vi "SetPoint.vi"(0 "Input":dbl, 1 "IAd(AI2)":dbl, 3 "I+(BI2)":bool, 4 "I-(BI1)":bool, 5 "Igrd(AI1)":dbl, 6 "ILL(AI3)":dbl=1.0, 7 "error in":errorcluster, 8 "ULL(AI4)":dbl=1.0, 9 "SetP Grad":dbl, 12 "IC(BI3)":bool, 14 "SetP UL":dbl, 15 "SetP LL":dbl) -> (23 "Output (AO1)":dbl, 27 "error out":errorcluster)   [LabVIEW 2022 SP3]
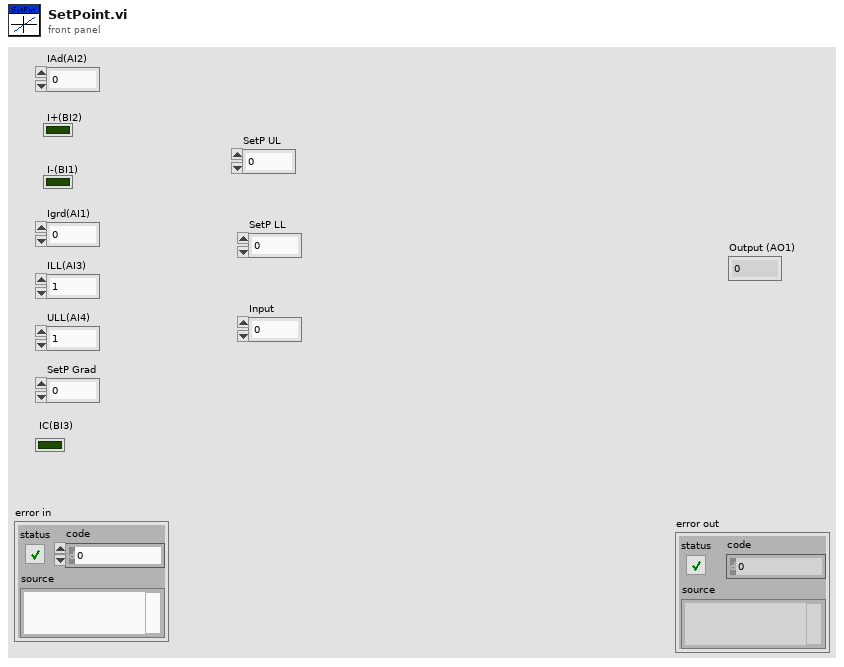
[diagram p1: front panel]
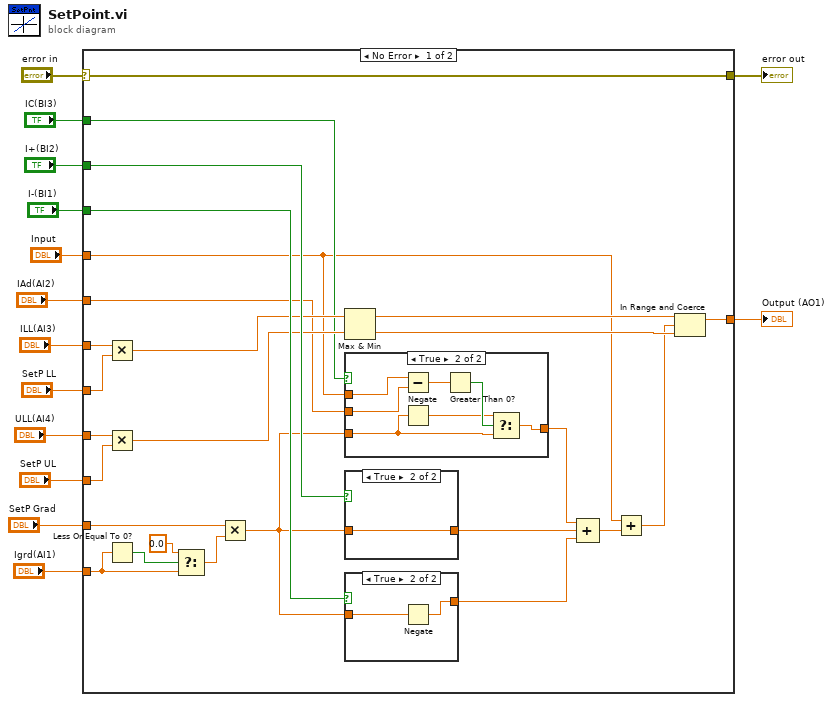
[diagram p0: block diagram]
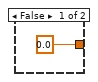
[diagram p2: hidden frame]
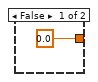
[diagram p3: hidden frame]
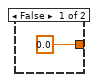
[diagram p4: hidden frame]
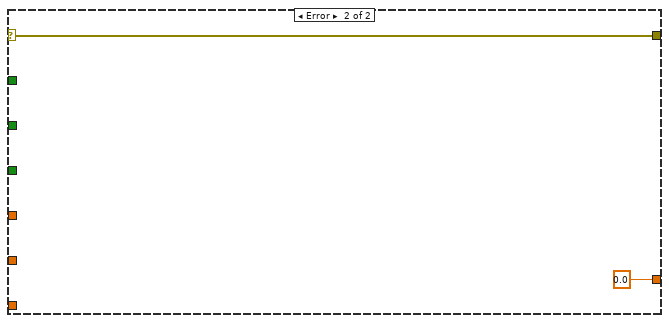
[diagram p5: hidden frame]
diagram:
  n1 = case shown="No Error" "error in" {
    selector: "error in" -> [w40 w54]
    tunnel: "Igrd(AI1)" -> [w36 _]
    tunnel: "IC(BI3)" -> [w18 _]
    tunnel: "IAd(AI2)" -> [w16 _]
    tunnel: [w19 0.0 ("IAd")] -> w11
    tunnel: "ILL(AI3)" -> [w28 _]
    tunnel: "ULL(AI4)" -> [w31 _]
    tunnel: [w40 w54] -> w7
    tunnel: "I+(BI2)" -> [w33 _]
    tunnel: "I-(BI1)" -> [w34 _]
    tunnel: "SetP Grad" -> [w39 _]
    tunnel: "SetP LL" -> [w26 _]
    tunnel: "SetP UL" -> [w25 _]
    tunnel: "Input" -> [w17 _]
    frame No Error {
      n2 = Multiply(x=w28, y=w26) -> (x*y=w32:dbl)
      n3 = Multiply(x=w31, y=w25) -> (x*y=w30:dbl)
      n4 = Less Or Equal To 0?(x=w36) -> (x <= 0?=w38:bool)
      n5 = Select(t=0.0, s=w38, f=w36) -> (s? t:f=w35:dbl)
      n6 = Multiply(x=w39, y=w35) -> (x*y=w21:dbl)
      n7 = Max & Min(x=w32, y=w30) -> (max(x,y)=w27:dbl, min(x,y)=w29:dbl)
      n8 = case shown="True" w18 {
        tunnel: w21 -> [_ w45]
        tunnel: w16 -> [_ w42]
        tunnel: [0.0 w44] -> w20
        tunnel: w17 -> [_ w43]
        frame False {
        }
        frame True {
          n9 = Subtract(x=w43, y=w42) -> (x-y=w47:dbl)
          n10 = Negate(x=w45) -> (-x=w46:dbl)
          n11 = Greater Than 0?(x=w47) -> (x > 0?=w48:bool)
          n12 = Select(t=w46, s=w48, f=w45) -> (s? t:f=w44:dbl)
        }
      }
      n13 = case shown="True" w33 {
        tunnel: w21 -> [_ w53]
        tunnel: [0.0 w53] -> w23
        frame False {
        }
        frame True {
        }
      }
      n14 = case shown="True" w34 {
        tunnel: w21 -> [_ w51]
        tunnel: [0.0 w50] -> w22
        frame False {
        }
        frame True {
          n15 = Negate(x=w51) -> (-x=w50:dbl)
        }
      }
      n16 = Compound Arithmetic op=ADD(w20, w23, w22) -> (w24:dbl)
      n17 = Add(x=w17, y=w24) -> (x+y=w15:dbl)
      n18 = In Range and Coerce(upper limit=w27, x=w15, lower limit=w29) -> (coerced(x)=w19:dbl)  [unwired: 1 out]
    }
    frame Error {
    }
  }
  "Output (AO1)" <- w11
  "error out" <- w7
